vi "ejercicicio1.vi"() -> ()   [LabVIEW 2017]
panel:
  out "Valor Encontrado":bool
  in  "Tiempo de espera en mS":dbl(knob) scale=0.0..1600.0
  out "Iteraciones":dbl
  out "Valor Aleatorio":dbl
  in  "Numero Buscado":dbl
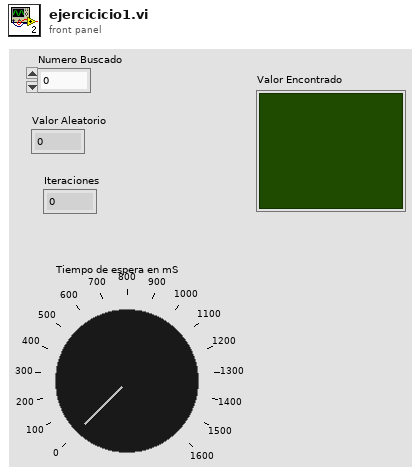
[diagram p1: front panel]
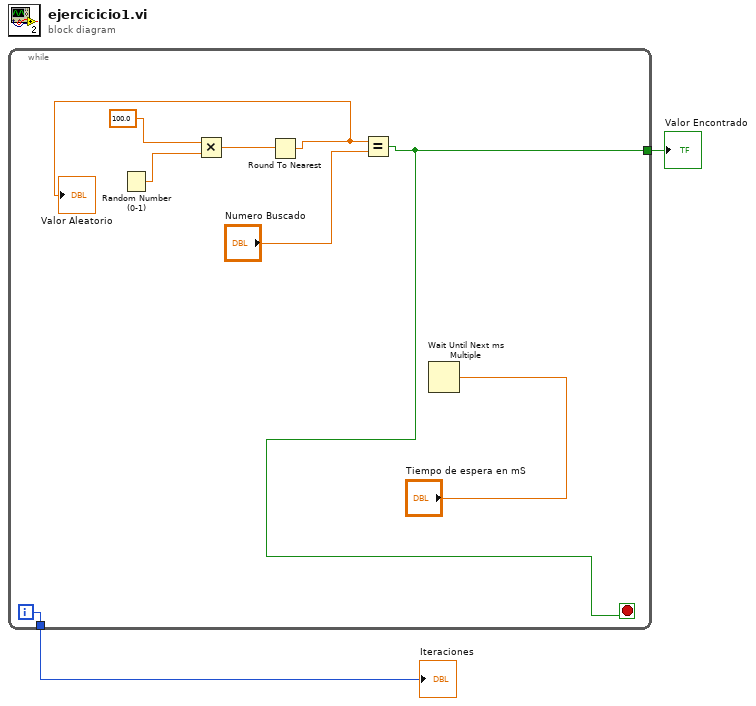
[diagram p0: block diagram]
diagram:
  n1 = while {
    tunnel: [w4] -> w2
    tunnel: [w3] -> w1
    i -> [w4]
    stop <- w3 stop-if-true
    n2 = Random Number (0-1)() -> (number: 0 to 1=w6:dbl)
    n3 = Multiply(x=100.0, y=w6) -> (x*y=w7:dbl)
    n4 = Round To Nearest(number=w7) -> (nearest integer value=w9:dbl)
    "Valor Aleatorio" <- w9
    n5 = Equal?(x=w9, y="Numero Buscado") -> (x = y?=w3:bool)
    n6 = Wait Until Next ms Multiple(millisecond multiple="Tiempo de espera en mS") -> ()  [unwired: 1 out]
  }
  "Iteraciones" <- w2
  "Valor Encontrado" <- w1
